vi "Deep Copy.vi"(8 "error in (no error)":errorcluster, 10 "Copy Actor In":refnum<class "System Actor.lvclass">, 11 "Root Actor in":refnum<class "Root Actor.lvclass">) -> (0 "error out":errorcluster, 2 "Coppied Actor Out":refnum<class "System Actor.lvclass">, 3 "Root Actor out":refnum<class "Root Actor.lvclass">)   [LabVIEW 2022 SP3, in "Root Actor.lvclass"]
uses:
  Root Actor.lvclass
  C:/Users/User/Desktop/Bussiness/Tricorn Re/Mandelbrot 4.0/General Library V2/Ancestor Class/Actor/System Actor/System Actor.lvclass
  System Actor/System Actor.lvclass
  Root Actor.lvclass/Root Actor.ctl
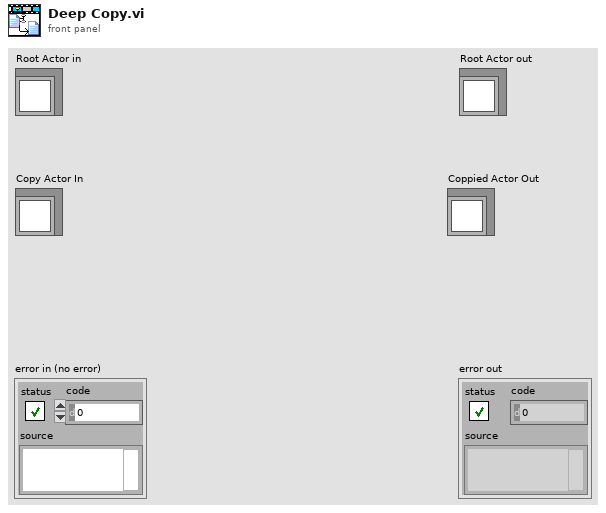
[diagram p1: front panel]
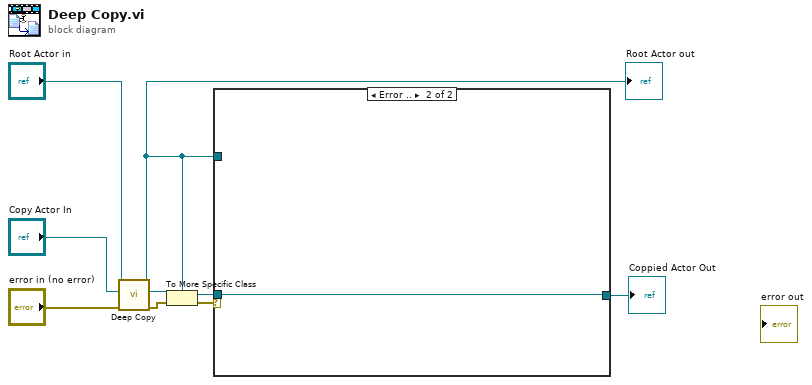
[diagram p0: block diagram]
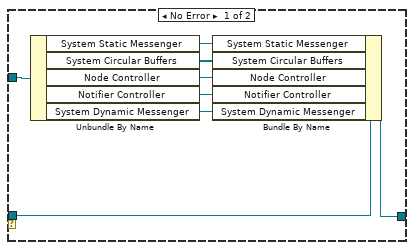
[diagram p2: hidden frame]
diagram:
  n1 = call-parent "Deep Copy.vi"("error in (no error)"="error in (no error)", "Copy Actor In"="Copy Actor In", "System Actor in"="Root Actor in") -> ("error out"=w4:errorcluster, "Coppied Actor Out"=w6:refnum<class "System Actor.lvclass">, "System Actor out"=w5:refnum<class "Root Actor.lvclass">)  [unwired: 6 in]
  "Root Actor out" <- w5
  n2 = To More Specific Class(target class=w5, reference=w6, error in=w4) -> (specific class reference=w2:refnum<class "Root Actor.lvclass">, error out=w3:errorcluster)
  n3 = case shown="Error .." w3 {
    tunnel: w5 -> [w17 _]
    tunnel: w2 -> [w16 w18]
    tunnel: [w10 w18] -> w1
    frame No Error {
      n4 = Unbundle By Name(w17) -> ("System Static Messenger"=w15:refnum<class "Messenger.lvclass">, "System Circular Buffers"=w14:refnum<class "Circular Buffer.lvclass">[], "Node Controller"=w13:refnum<class "Node Controller.lvclass">, "Notifier Controller"=w12:refnum<class "Notifier Controller.lvclass">, "System Dynamic Messenger"=w11:refnum<class "Messenger.lvclass">)
      n5 = Bundle By Name(cluster=w16, "System Static Messenger"=w15, "System Circular Buffers"=w14, "Node Controller"=w13, "Notifier Controller"=w12, "System Dynamic Messenger"=w11) -> (w10:refnum<class "Root Actor.lvclass">)
    }
    frame Error {
    }
  }
  "Coppied Actor Out" <- w1
